vi "Get SMO HAL Type.vi"(8 "error in (no error)":errorcluster, 11 "Instrument in":refnum<class "Instrument.lvclass">) -> (0 "error out":errorcluster, 2 "Dependencies.HAL":refnum<class "HAL.lvclass">, 3 "Instrument out":refnum<class "Instrument.lvclass">)   [LabVIEW 2019, in "Instrument.lvclass"]
doc: "Override this VI to return the type of RemoteControl process used by your Instrument. The default is RemoteControl.ZMQ"
uses:
  Instrument.lvclass
  subsystems/HAL/HAL.lvclass
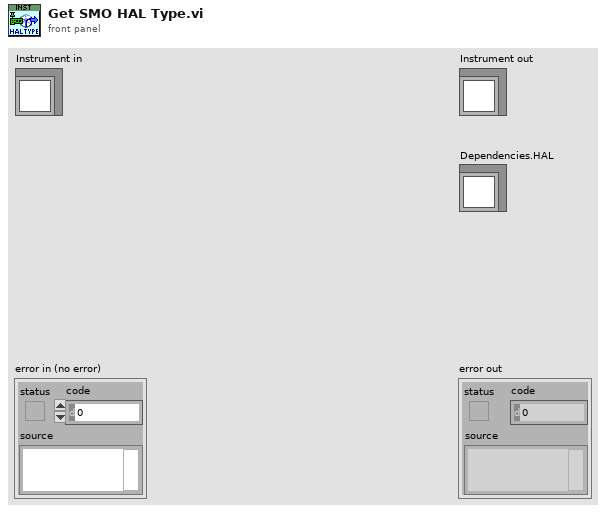
[diagram p1: front panel]
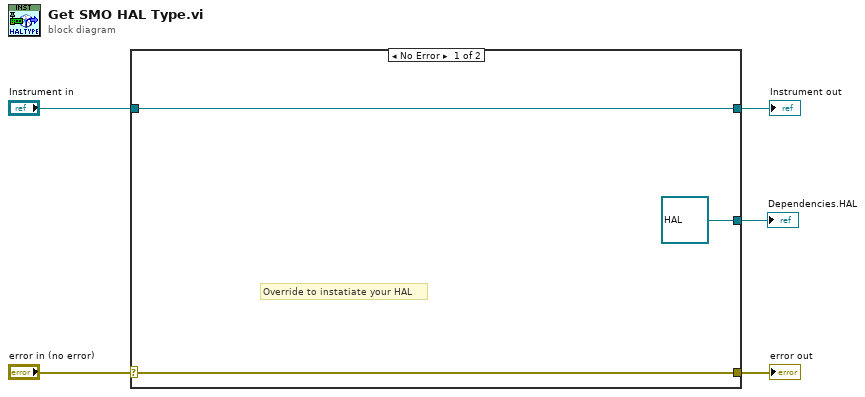
[diagram p0: block diagram]
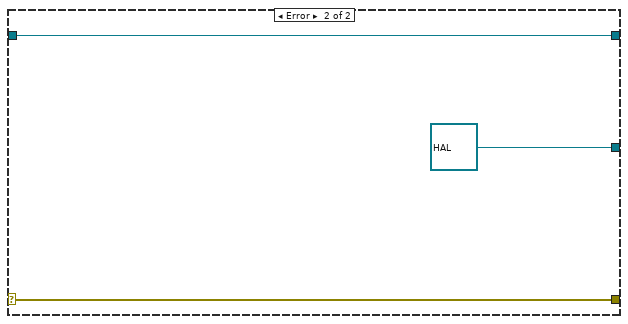
[diagram p2: hidden frame]
diagram:
  n1 = case shown="No Error" "error in (no error)" {
    selector: "error in (no error)" -> [w8 w11]
    tunnel: [w8 w11] -> w4
    tunnel: [w7 w10] -> w2
    tunnel: "Instrument in" -> [w7 w10]
    tunnel: [refnum<class "HAL.lvclass"> refnum ("HAL.lvclass") refnum<class "HAL.lvclass"> refnum ("HAL.lvclass")] -> w1
    frame No Error {
      # "Override to instatiate your HAL"
    }
    frame Error {
    }
  }
  "error out" <- w4
  "Instrument out" <- w2
  "Dependencies.HAL" <- w1
